vi "Apagar_led_cam.vi"(8 "error in (no error)":errorcluster, 11 "DNVideoX":refnum<k7>(container)) -> (0 "error out":errorcluster, 3 "reference out":refnum<k7>)   [LabVIEW 2019]
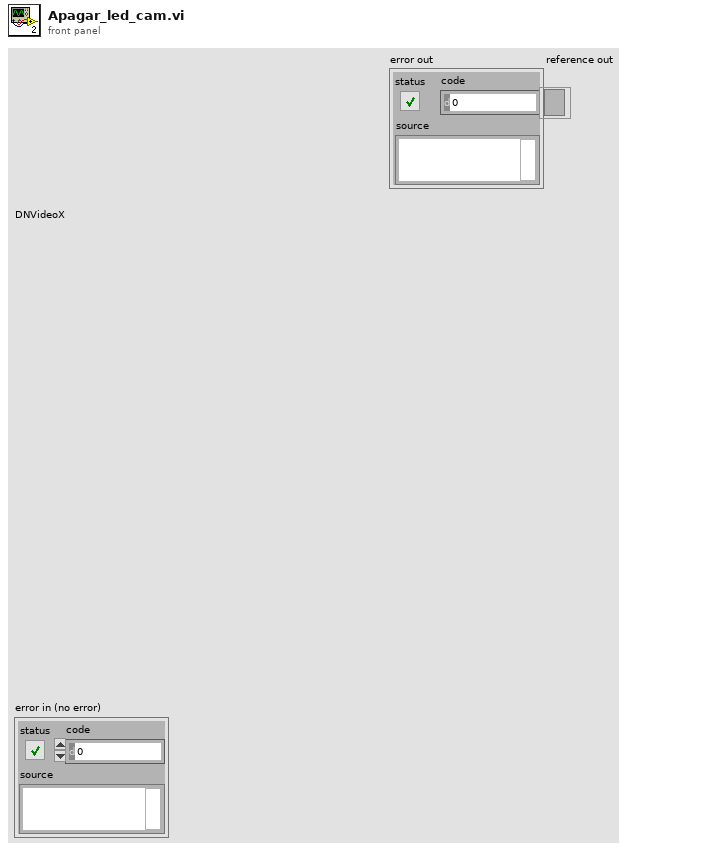
[diagram p1: front panel]
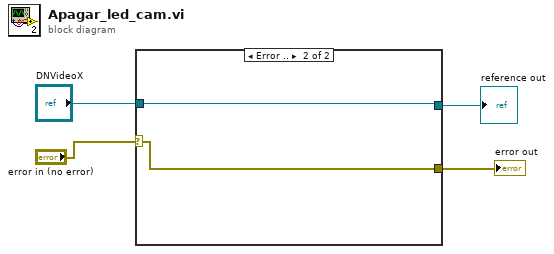
[diagram p0: block diagram]
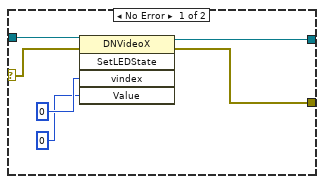
[diagram p2: hidden frame]
diagram:
  n1 = case shown="Error .." "error in (no error)" {
    selector: "error in (no error)" -> [w5 w11]
    tunnel: [w8 w11] -> w4
    tunnel: [w7 w12] -> w3
    tunnel: "DNVideoX" -> [w6 w12]
    frame No Error {
      n2 = invoke class="DNVideoX" method="SetLEDState"(reference=w6, error in=w5, "vindex"=0, "Value"=0) -> (reference out=w7:refnum<k7>, error out=w8:errorcluster)  [unwired: 1 in, 3 out]
    }
    frame Error {
    }
  }
  "error out" <- w4
  "reference out" <- w3
